vi "Main.vi"() -> ()   [LabVIEW 2014]
panel:
  out "Output":string
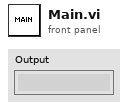
[diagram p1: front panel]
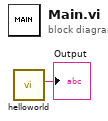
[diagram p0: block diagram]
diagram:
  n1 = call "helloworld.vi"() -> ("Output"=→"Output":string)  [unwired: 11 in]
